vi "Galvo Offset AE v1.vi"(2 "Galvo 1 Offset In":dbl format="%#_13g", 3 "Action":enum16{"Read", "Write"}(ring)) -> (0 "Galvo 2 Offset Out":dbl, 1 "Galvo 1 Offset Out":dbl format="%#_13g")   [LabVIEW 2014]
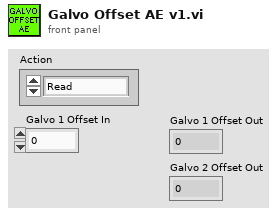
[diagram p1: front panel]
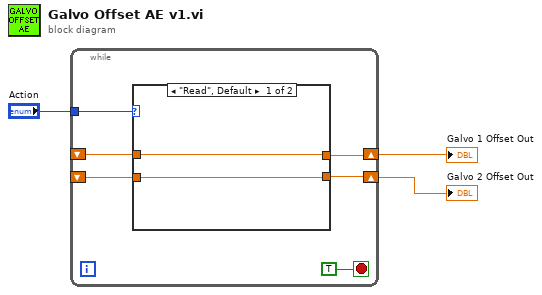
[diagram p0: block diagram]
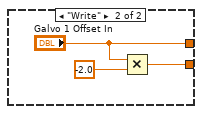
[diagram p2: hidden frame]
diagram:
  n1 = while {
    shift-right: [w7] -> w2
    shift-left: _ -> [w6]
    tunnel: "Action" -> [w8]
    shift-right: [w5] -> w1
    shift-left: _ -> [w4]
    stop <- TRUE stop-if-true
    n2 = case shown="\"Read\", Default" w8 {
      tunnel: [w11 "Galvo 1 Offset In"] -> w7
      tunnel: w6 -> [w11 _]
      tunnel: [w10 w12] -> w5
      tunnel: w4 -> [w10 _]
      frame "Read", Default {
      }
      frame "Write" {
        n3 = Multiply(x="Galvo 1 Offset In", y=-2.0) -> (x*y=w12:dbl)
      }
    }
  }
  "Galvo 1 Offset Out" <- w2
  "Galvo 2 Offset Out" <- w1
